vi "Pause.vi"(8 "error in (no error)":errorcluster, 11 "FLOM Settings in":T1={"VISA resource name"="", "Simulated?"=FALSE, "Pump Number"=1.0} {"Pump Number" min=1.0 max=20.0 step=1.0}) -> (0 "error out":errorcluster, 1 "Connection Error":bool, 3 "FLOM Settings out":T1={"VISA resource name"="", "Simulated?"=FALSE, "Pump Number"=1.0} {"Pump Number" min=1.0 max=20.0 step=1.0})   [LabVIEW 2018, in "FLOM Pump.lvlib"]
uses:
  FLOM Pump.lvlib
  Settings Cluster.ctl
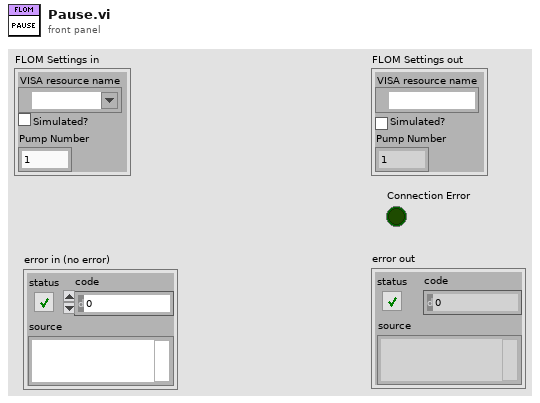
[diagram p1: front panel]
types:
  T1 = typedef "FLOM Pump.lvlib/Settings Cluster.ctl" = cluster{"VISA resource name":refnum<visa-resource-name>, "Simulated?":bool, "Pump Number":dbl}
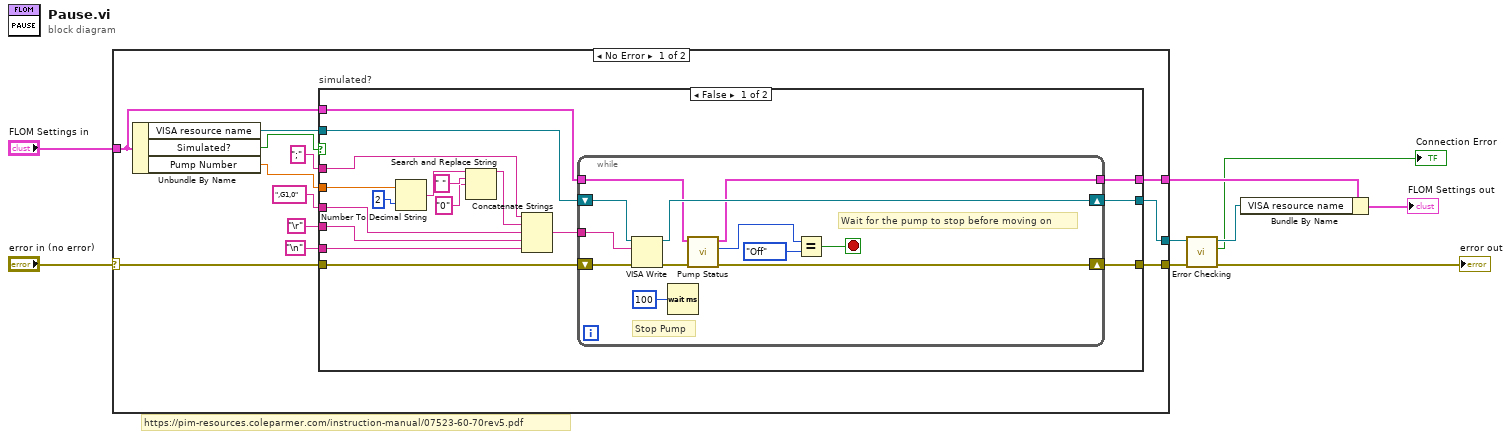
[diagram p0: block diagram]
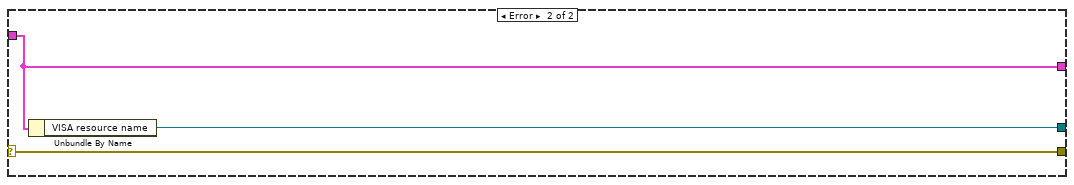
[diagram p3: hidden frame]
diagram:
  # "https://pim-resources.coleparmer.com/instruction-manual/07523-60-70rev5.pdf"
  n1 = case shown="No Error" "error in (no error)" {
    selector: "error in (no error)" -> [w19 w56]
    tunnel: [w15 w55] -> w9
    tunnel: "FLOM Settings in" -> [w16 w55]
    tunnel: [w18 w54] -> w6
    tunnel: [w17 w56] -> w7
    frame No Error {
      n2 = Unbundle By Name(w16) -> ("VISA resource name"=w21:refnum<visa-resource-name>, "Simulated?"=w20:bool, "Pump Number"=w14:dbl)
      n3 = case "simulated?" shown="False" w20 {
        tunnel: [w36 w53] -> w18
        tunnel: w21 -> [w38 w53]
        tunnel: w19 -> [w37 w52]
        tunnel: [w35 w52] -> w17
        tunnel: w16 -> [w34 w51]
        tunnel: [w33 w51] -> w15
        tunnel: w14 -> [w27 _]
        tunnel: "\n" -> [w23 _]
        tunnel: "\r" -> [w24 _]
        tunnel: ",G1,0" ("string") -> [w25 _]
        tunnel: ";" ("string") -> [w26 _]
        frame False {
          n4 = Number To Decimal String(number=w27, width (-)=i16 2) -> (decimal integer string=w31:string)
          n5 = Search and Replace String(input string=w31, search string=" ", replace string="0" ("replace string (\"\")")) -> (result string=w32:string)  [unwired: 5 in, 3 out]
          n6 = Concatenate Strings(w26, w32, w25, w24, w23) -> (w22:string)
          n7 = while {
            shift-right: [w48] -> w36
            shift-left: w38 -> [w50]
            shift-right: [w43] -> w35
            shift-left: w37 -> [w49]
            tunnel: w34 -> [w46]
            tunnel: [w45] -> w33
            tunnel: w22 -> [w39]
            stop <- w41 stop-if-true
            # "Wait for the pump to stop before moving on"
            # "Stop Pump"
            n8 = VISA Write(VISA resource name=w50, write buffer=w39, error in (no error)=w49) -> (VISA resource name out=w48:refnum<visa-resource-name>, error out=w44:errorcluster)  [unwired: 1 out]
            n9 = Wait (ms)(milliseconds to wait=u32 100) -> ()  [unwired: 1 out]
            n10 = call "Pump Status.vi"("error in (no error)"=w44, "FLOM Settings In"=w46) -> ("error out"=w43:errorcluster, "Pump On?"=w42:enum16{"Off", "On", "Not Initialized"}, "FLOM Settings Out"=w45:T1)  [unwired: 4 in, 3 out]
            n11 = Equal?(x=w42, y=enum16{"Off", "On", "Not Initialized"}."Off") -> (x = y?=w41:bool)
          }
        }
        frame True {
        }
      }
    }
    frame Error {
      n12 = Unbundle By Name(w55) -> ("VISA resource name"=w54:refnum<visa-resource-name>)
    }
  }
  n13 = call "Error Checking.vi"("error in (no error)"=w7, "VISA resource name"=w6) -> ("error out"=→"error out":errorcluster, "Connection Error"=→"Connection Error":bool, "VISA resource name"=w8:refnum<visa-resource-name>)  [unwired: 7 in]
  n14 = Bundle By Name(cluster=w9, "VISA resource name"=w8) -> (→"FLOM Settings out":T1)
